vi "PFI-28000-Base_Create.vi"(0 "PFI-28000-Base in":refnum<class "PFI-28000-Base.lvclass">, 5 "Parent":refnum<class "PFI-28000-Base.lvclass">, 11 "error in (no error)":errorcluster) -> (4 "PFI-28000-Base out":refnum<class "PFI-28000-Base.lvclass">, 15 "error out":errorcluster)   [LabVIEW 2017, in "PFI-28000-Base.lvclass"]
uses:
  PFI-28000-Base.lvclass
  Overload/PFI-28000-Overload.lvclass
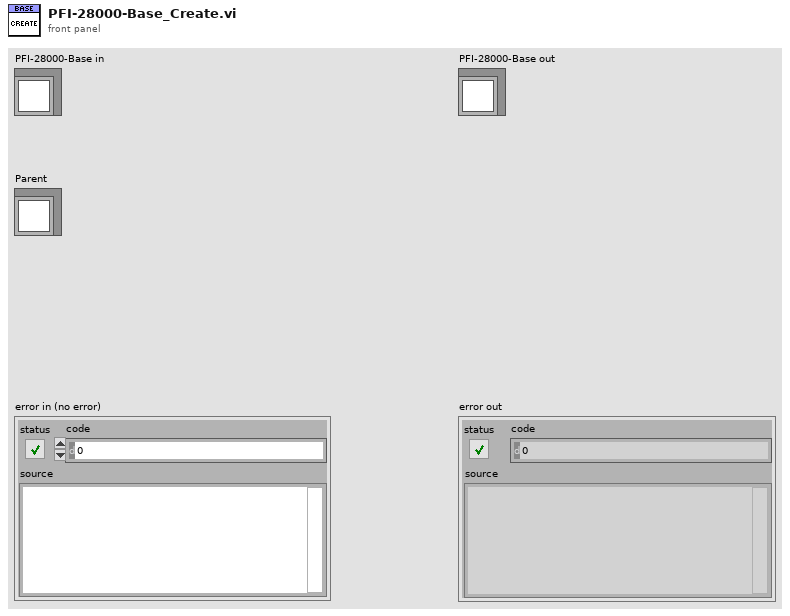
[diagram p1: front panel]
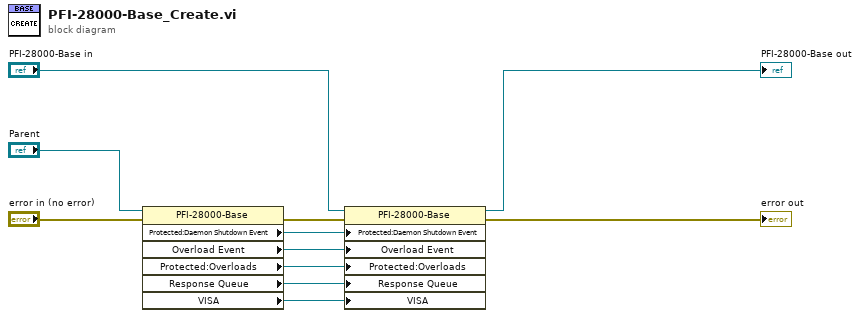
[diagram p0: block diagram]
diagram:
  n1 = property class="PFI-28000-Base"(reference="Parent", error in="error in (no error)") -> (error out=w9:errorcluster, "Protected:Daemon Shutdown Event"=w7:refnum<user-event>, "Overload Event"=w6:refnum<user-event>, "Protected:Overloads"=w5:refnum<data-value>, "Response Queue"=w4:refnum<queue>, "VISA"=w3:refnum<visa-resource-name>)  [unwired: 1 out]
  n2 = property class="PFI-28000-Base"(reference="PFI-28000-Base in", error in=w9, "Protected:Daemon Shutdown Event"=w7, "Overload Event"=w6, "Protected:Overloads"=w5, "Response Queue"=w4, "VISA"=w3) -> (reference out=→"PFI-28000-Base out":refnum<class "PFI-28000-Base.lvclass">, error out=→"error out":errorcluster)
